vi "Write_instrument-type.vi"(8 "error in (no error)":errorcluster, 10 "instrument type":u16(ring) items=["Spectrometer", "TempController", "PGaugeController", "SwitchController", "Generic"], 11 "instrument in":refnum<class "instrument.lvclass">) -> (0 "error out":errorcluster, 3 "instrument out":refnum<class "instrument.lvclass">)   [LabVIEW 2018, in "instrument.lvclass"]
uses:
  instrument.lvclass
  instrument.lvclass/instrument.ctl
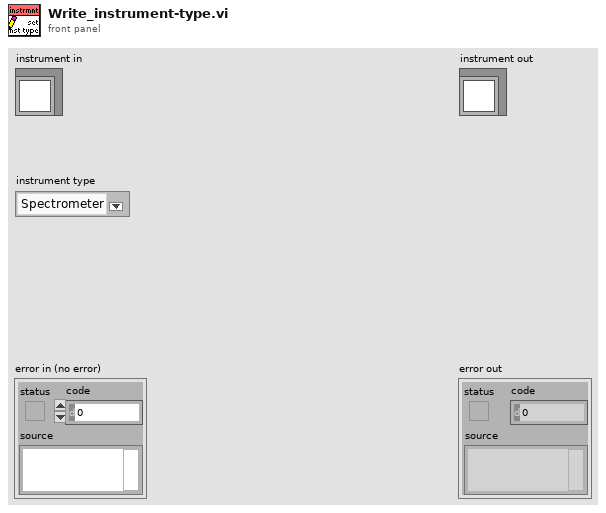
[diagram p1: front panel]
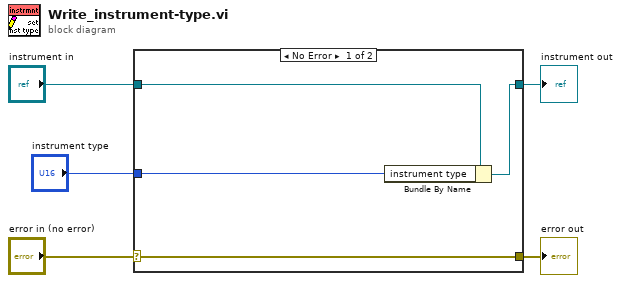
[diagram p0: block diagram]
diagram:
  n1 = case shown="No Error" "error in (no error)" {
    selector: "error in (no error)" -> [w9 w10]
    tunnel: [w9 w10] -> w4
    tunnel: [w7 w11] -> w2
    tunnel: "instrument in" -> [w8 w11]
    tunnel: "instrument type" -> [w6 _]
    frame No Error {
      n2 = Bundle By Name(cluster=w8, "instrument type"=w6) -> (w7:refnum<class "instrument.lvclass">)
    }
    frame Error {
    }
  }
  "error out" <- w4
  "instrument out" <- w2
